vi "new Reserver Filter.vi"(10 "Reserver Ref in":T1 format="%.0x") -> (2 "reserver filter out":refnum<class "Filter.lvclass">)   [LabVIEW 2016, in "Reserver Filter.lvclass"]
uses:
  Reserver Filter.lvclass
  Filter Parent/Filter.lvclass
  <vilib>/NI Veristand/Custom Device API/Custom Device Item Ref.ctl
  C:/github/VeriStand-FPGA-Resource-Manager/Source/Filters/Filter Parent/Filter.lvclass
  Reserver Filter.lvclass/Reserver Filter.ctl
  <vilib>/NI Veristand/Custom Device API/Custom Device API.lvlib
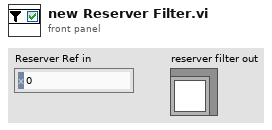
[diagram p1: front panel]
types:
  T1 = typedef "Custom Device API.lvlib/Custom Device Item Ref.ctl" = u64
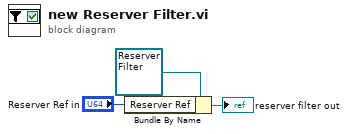
[diagram p0: block diagram]
diagram:
  n1 = Bundle By Name(cluster=refnum<class "Reserver Filter.lvclass"> refnum ("Reserver Filter in"), "Reserver Ref"="Reserver Ref in") -> (→"reserver filter out":refnum<class "Reserver Filter.lvclass">)
